vi "Write Element of Paths.vi"(8 "error in (no error)":errorcluster, 10 "Path Settings.lvclass":refnum<class "Path Settings.lvclass">, 11 "Setting Database in":refnum<class "Setting Database.lvclass">) -> (0 "error out":errorcluster, 3 "Setting Database out":refnum<class "Setting Database.lvclass">)   [LabVIEW 2020, in "Setting Database.lvclass"]
uses:
  Setting Database.lvclass
  Path Settings/Path Settings.lvclass
  Setting Database.lvclass/Setting Database.ctl
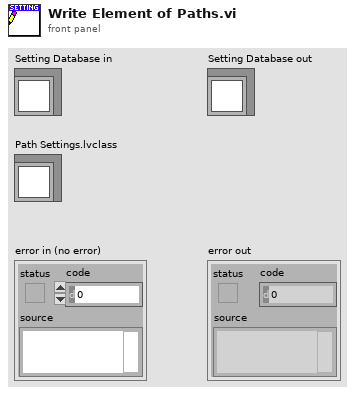
[diagram p1: front panel]
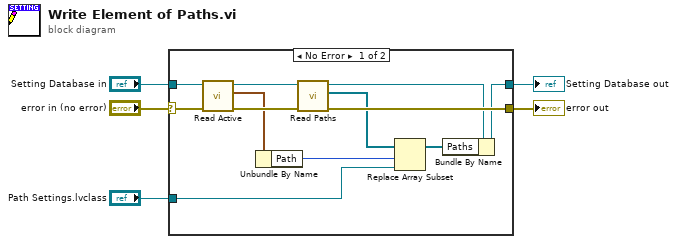
[diagram p0: block diagram]
diagram:
  n1 = case shown="No Error" "error in (no error)" {
    selector: "error in (no error)" -> [w16 w19]
    tunnel: [w15 w19] -> w4
    tunnel: [w13 w18] -> w2
    tunnel: "Setting Database in" -> [w9 w18]
    tunnel: "Path Settings.lvclass" -> [w6 _]
    frame No Error {
      n2 = call "Read Active.vi"("error in (no error)"=w16, "Setting Database in"=w9) -> ("error out"=w17:errorcluster, "Active"=w8:cluster{"Path":i32}, "Setting Database out"=w10:refnum<class "Setting Database.lvclass">)  [unwired: 7 in]
      n3 = Unbundle By Name(w8) -> ("Path"=w7:i32)
      n4 = call "Read Paths.vi"("error in (no error)"=w17, "Setting Database in"=w10) -> ("error out"=w15:errorcluster, "Paths"=w11:refnum<class "Path Settings.lvclass">[], "Setting Database out"=w12:refnum<class "Setting Database.lvclass">)  [unwired: 7 in]
      n5 = Replace Array Subset(array=w11, new element=w6, index=w7) -> (w14:refnum<class "Path Settings.lvclass">[])
      n6 = Bundle By Name(cluster=w12, "Paths"=w14) -> (w13:refnum<class "Setting Database.lvclass">)
    }
    frame Error {
    }
  }
  "error out" <- w4
  "Setting Database out" <- w2
